vi "fake_read_onepixel.vi"(1 "pixel counter":u8) -> (0 "input cluster":T1)   [LabVIEW 2010]
uses:
  common_typedefs/channels_cluster.ctl
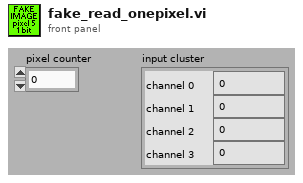
[diagram p1: front panel]
types:
  T1 = typedef "channels_cluster.ctl" = cluster{"channel 0":u32, "channel 1":u32, "channel 2":u32, "channel 3":u32}
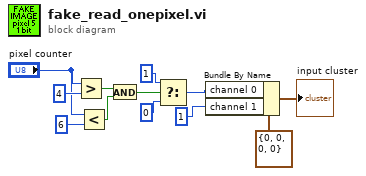
[diagram p0: block diagram]
diagram:
  n1 = Greater?(x="pixel counter", y=u8 4) -> (0:w3:bool)
  n2 = Less?(x="pixel counter", y=u8 6) -> (x < y?=w2:bool)
  n3 = And(x=w3, y=w2) -> (x .and. y?=w1:bool)
  n4 = Select(t=u16 1 ("y"), s=w1, f=u16 0) -> (s? t:f=w10:u16)
  n5 = Bundle By Name(cluster=T1 {"channel 0"=0, "channel 1"=0, "channel 2"=0, "channel 3"=0} ("input cluster"), "channel 0"=w10, "channel 1"=u16 1 ("f")) -> (→"input cluster":T1)
